vi "布尔转OKNG.vi"(1 "数组":bool[](array[boolean])) -> (0 "数组 out":string[](array[string]))   [LabVIEW 2020]
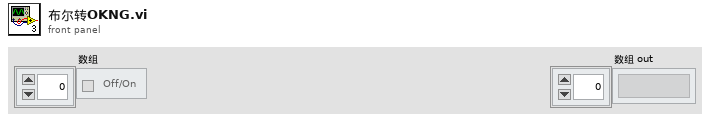
[diagram p1: front panel]
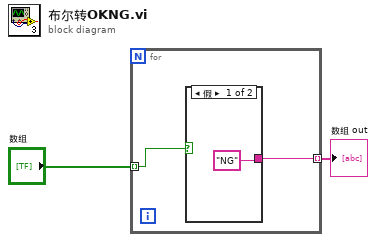
[diagram p0: block diagram]
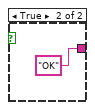
[diagram p2: hidden frame]
diagram:
  n1 = for {
    tunnel: "数组" -> [w4] mode=indexing
    tunnel: [w3] -> w1 mode=indexing
    n2 = case shown="假" w4 {
      tunnel: ["NG" "OK"] -> w3
      frame False {
      }
      frame True {
      }
    }
  }
  "数组 out" <- w1
